vi "Parent Class Teardown.vi"(8 "error in (no error)":errorcluster, 11 "class string":refnum<class "Parent.lvclass">) -> (0 "error out":errorcluster, 2 "String Data":string)   [LabVIEW 2023]
doc: "This VI accesses to Parent.ctl, the data member of Parent.lvclass, by calling the Read String Data VI.\n\nUsed this VI as a teardown VI for the Add Prefix.lvtest test."
uses:
  Parent.lvclass
panel:
  # "Overview:\nThis VI accesses to Parent.ctl, the data member of Parent.lvclass, by calling the Read String Data VI.\nUsed this VI as a teardown VI for the Add Prefix.lvtest test."
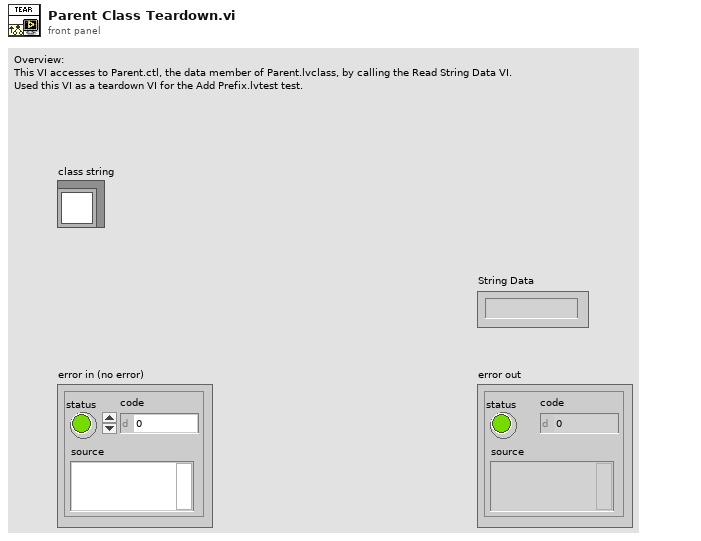
[diagram p1: front panel]
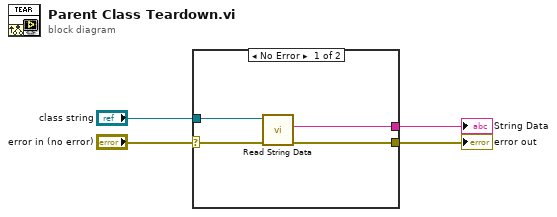
[diagram p0: block diagram]
diagram:
  n1 = case shown="No Error" "error in (no error)" {
    selector: "error in (no error)" -> [w5 w9]
    tunnel: "class string" -> [w8 _]
    tunnel: [w7 _] -> w3
    tunnel: [w6 w9] -> w2
    frame No Error {
      n2 = call-dynamic "Read String Data.vi"("error in (no error)"=w5, "class string in"=w8) -> ("error out"=w6:errorcluster, "String Data"=w7:string)  [unwired: 7 in, 1 out]
    }
    frame Error {
    }
  }
  "String Data" <- w3
  "error out" <- w2
